vi "ArdnoFeed.vi"(0 "LINX Resource":T2={"IO"=enum."Remote", "Interface"=enum."Serial", "LINX Device Config"={"Interface"=enum."Serial", "COM Port"="COM13", "TCP Configuration"={"IP Address"="", "Port"=0}, "Device Family"=1, "Device ID"=1, "Device Name"="myRIO-1900", "TCP Ref"=refnum, "Channels"={"DI"=[0, 1, 2, 3, 4, 5, 6, 7, 8, 9, 10, 11, 12, 13, 14, 15, 16, 17, 18, 19, 20, 21, 22, 23, 24, 25, 26, 27, 28, 29, 30, 31, 32, 33, 34, 35, 36, 37, 38, 39, 40, 41, 42, 43, 44, 45, 46], "DO"=[0, 1, 2, 3, 4, 5, 6, 7, 8, 9, 10, 11, 12, 13, 14, 15, 16, 17, 18, 19, 20, 21, 22, 23, 24, 25, 26, 27, 28, 29, 30, 31, 32, 33, 34, 35, 36, 37, 38, 39, 40, 41, 42, 43, 44, 45, 46], "AI"=[0, 1, 2, 3, 4, 5, 6, 7, 8, 9, 10, 11], "AO"=[], "PWM"=[3, 5, 6, 9, 10], "QE"=[], "UART"=[0, 1], "I2C 2"=[0], "SPI"=[0], "CAN"=[], "Servo"=[], "AI Ref (V)"=0.0, "AI Resolution (Bits)"=0, "AO Ref (V)"=0.0, "AO Resolution (Bits)"=0}}}, 1 "Single / Multiring?":bool, 5 "Channel":u32, 7 "Ring":u16, 9 "Feed Cycles":i32, 11 "error in (no error)":errorcluster, 12 "All Rings":bool) -> (4 "LINX Resource out":T2, 6 "Elapsed [ms]":u32, 15 "error out":errorcluster)   [LabVIEW 2018, in "Arduino.lvlib"]
uses:
  Arduino.lvlib
  <vilib>/MakerHub/LINX/Private/Type Defs/LINX Ref.ctl
  <vilib>/MakerHub/LINX/Private/Type Defs/Platform.ctl
  <vilib>/MakerHub/LINX/Private/Type Defs/Interface.ctl
  <vilib>/MakerHub/LINX/Private/Device/Type Defs/LINX Device Config.ctl
  <vilib>/MakerHub/LINX/Private/Device/Type Defs/TCP Config.ctl
  <vilib>/MakerHub/LINX/Private/Device/Type Defs/Channels.ctl
  <vilib>/MakerHub/LINX/Public/Peripherals/Digital/Digital Write N Chans.vi
  <vilib>/MakerHub/LINX/Private/Local IO/LinxDigitalWrite.vi
  <vilib>/MakerHub/LINX/Public/Utilities/Check Channel.vi
  <vilib>/MakerHub/LINX/Private/Utilties/Generate Error.vi
  <vilib>/MakerHub/LINX/LMH-LINX.lvlib
  <vilib>/MakerHub/LINX/Private/Device/Device.lvlib
panel:
  in  "ValveManualCluster":T1
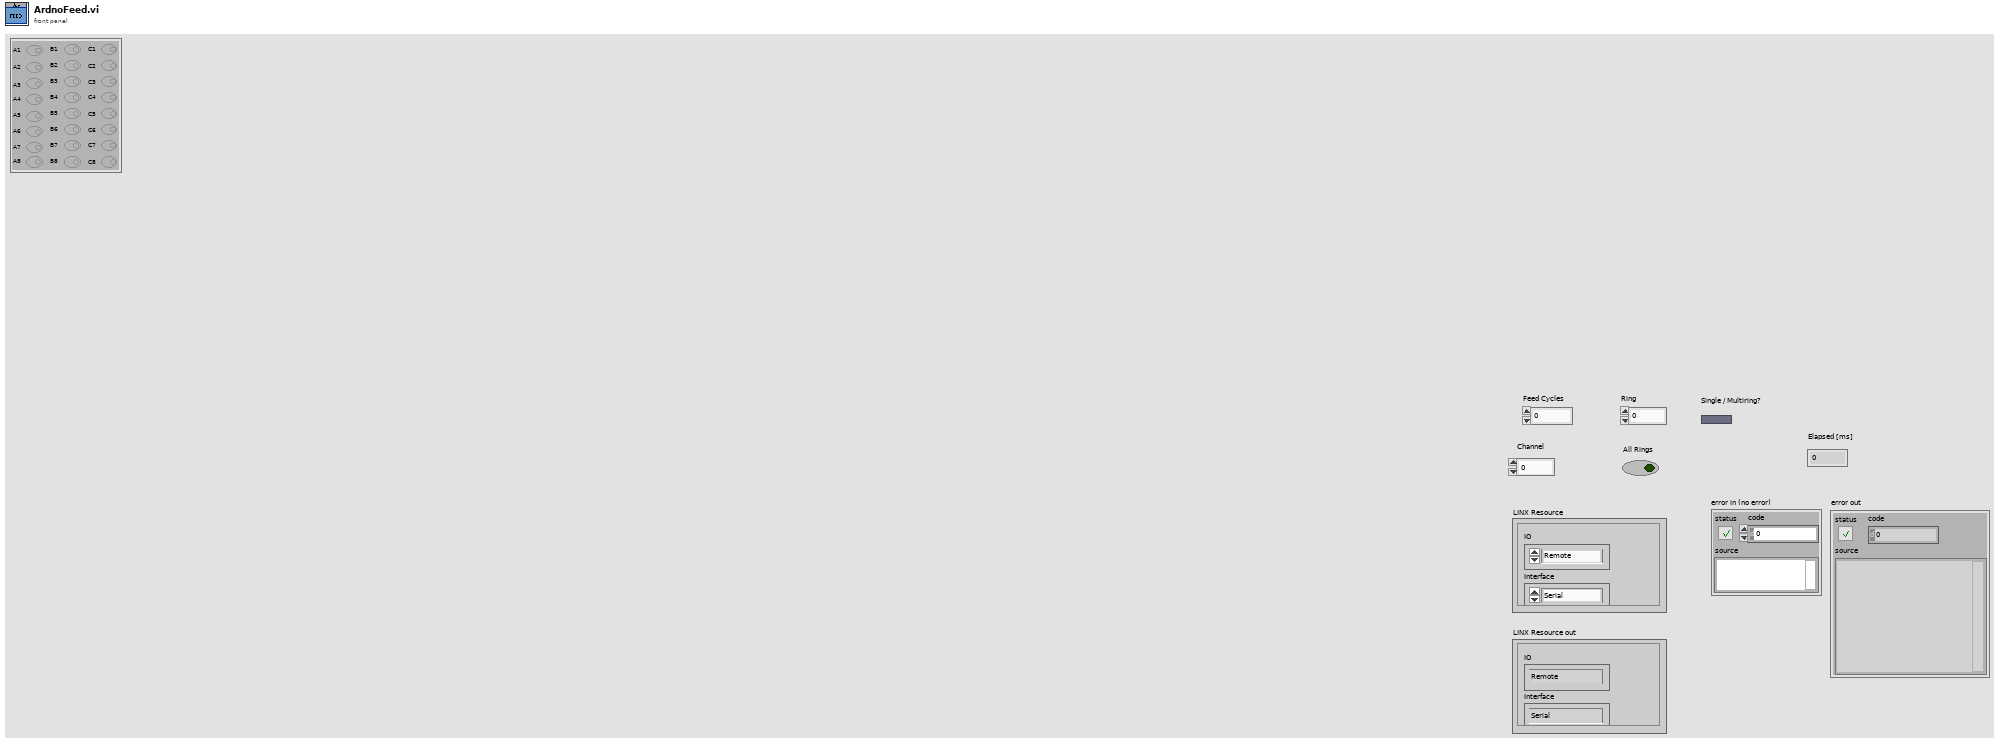
[diagram p1: front panel]
types:
  T1 = cluster{"C8":bool, "C7":bool, "C6":bool, "C5":bool, "C4":bool, "C3":bool, "C2":bool, "C1":bool, "B8":bool, "B7":bool, "B6":bool, "B5":bool, "B4":bool, "B3":bool, "B2":bool, "B1":bool, "A8":bool, "A7":bool, "A6":bool, "A5":bool, "A4":bool, "A3":bool, "A2":bool, "A1":bool}
  T2 = typedef "LMH-LINX.lvlib/LINX Ref.ctl" = cluster{"IO":T3, "Interface":T4, "LINX Device Config":T5}
  T3 = typedef "LMH-LINX.lvlib/Platform.ctl" = enum16{"Remote", "Local"}
  T4 = typedef "LMH-LINX.lvlib/Interface.ctl" = enum16{"Serial", "TCP"}
  T5 = typedef "LMH-LINX.lvlib/Device.lvlib/LINX Device Config.ctl" = cluster{"Interface":T4, "COM Port":refnum<visa-resource-name>, "TCP Configuration":T6, "Device Family":u8, "Device ID":u8, "Device Name":string, "TCP Ref":refnum<k5>, "Channels":T7}
  T6 = typedef "LMH-LINX.lvlib/Device.lvlib/TCP Config.ctl" = cluster{"IP Address":string, "Port":u16}
  T7 = typedef "LMH-LINX.lvlib/Channels.ctl" = cluster{"DI":u8[], "DO":u8[], "AI":u8[], "AO":u8[], "PWM":u8[], "QE":u8[], "UART":u8[], "I2C 2":u8[], "SPI":u8[], "CAN":u8[], "Servo":u8[], "AI Ref (V)":dbl, "AI Resolution (Bits)":u8, "AO Ref (V)":dbl, "AO Resolution (Bits)":u8}
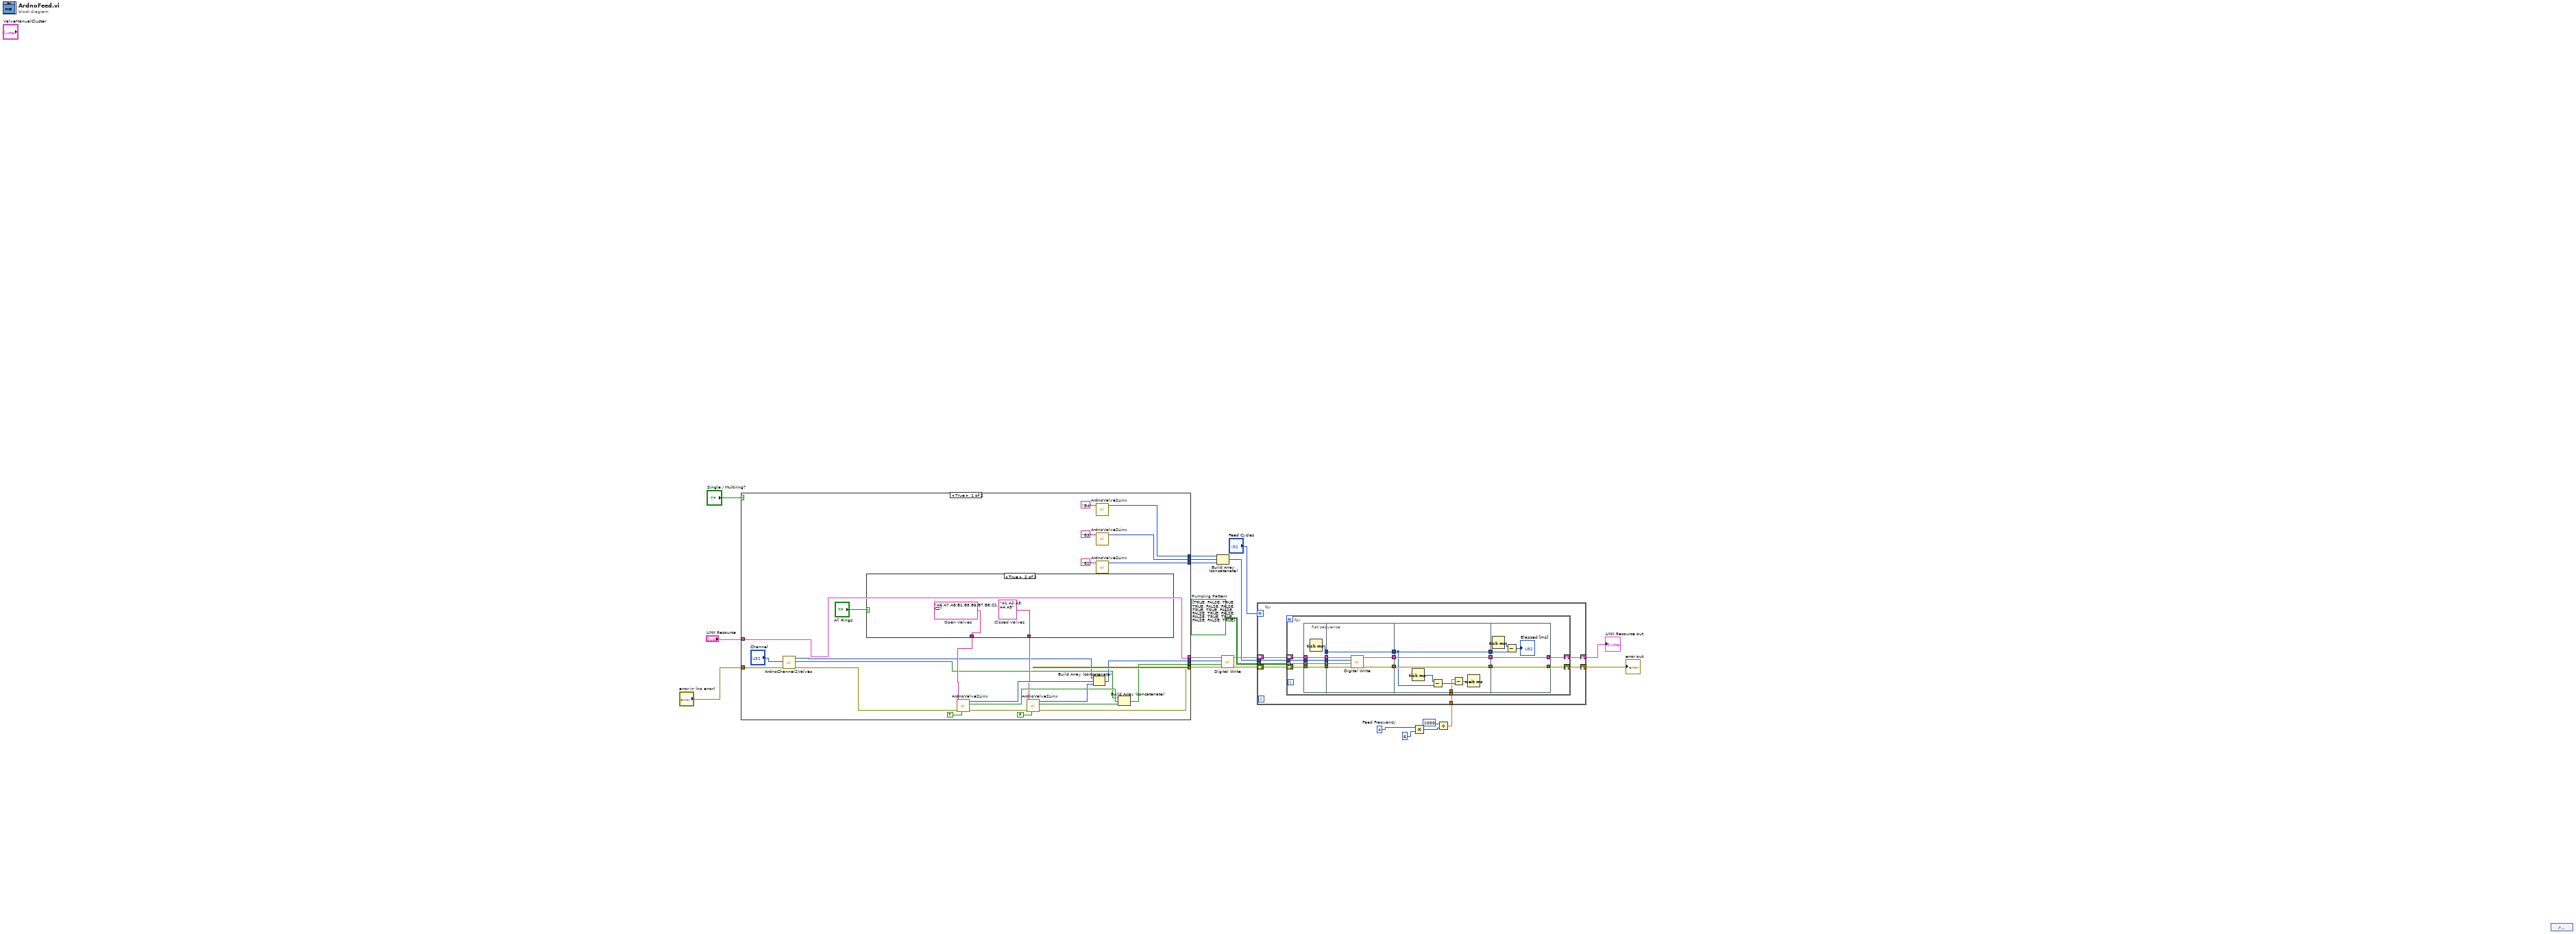
[diagram p0: block diagram]
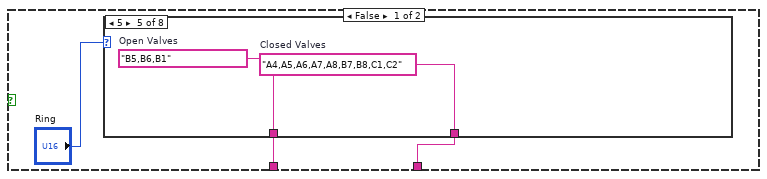
[diagram p2: hidden frame]
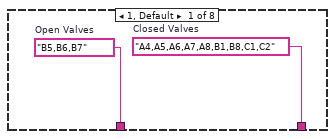
[diagram p3: hidden frame]
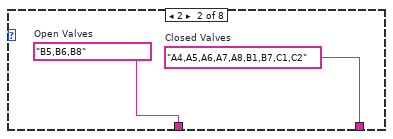
[diagram p4: hidden frame]
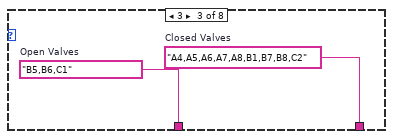
[diagram p5: hidden frame]
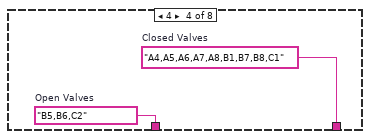
[diagram p6: hidden frame]
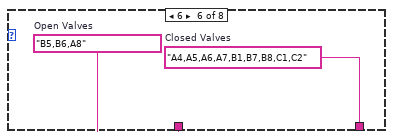
[diagram p7: hidden frame]
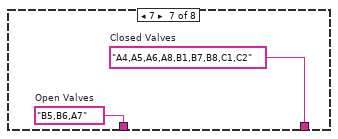
[diagram p8: hidden frame]
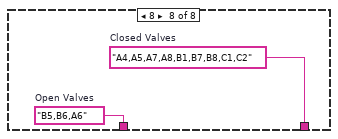
[diagram p9: hidden frame]
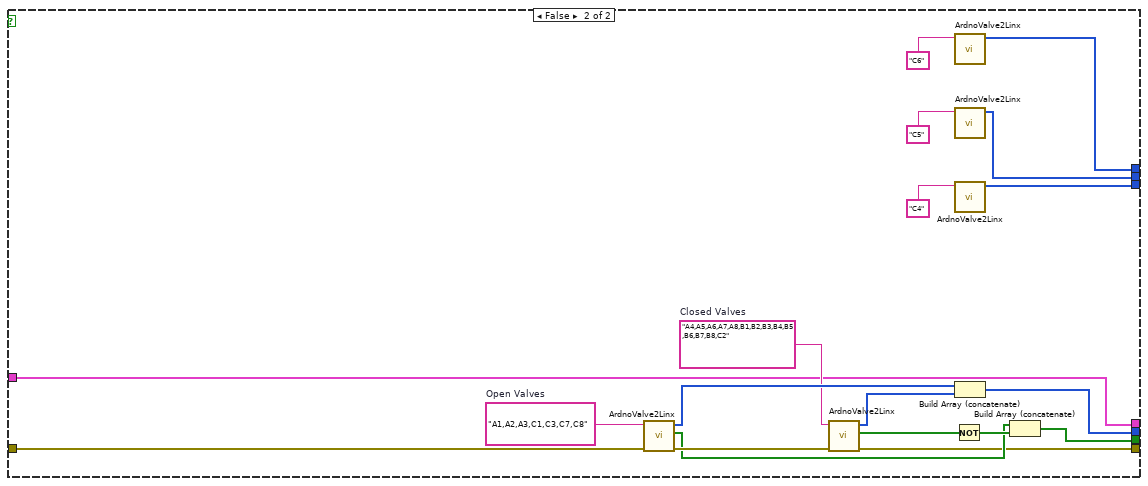
[diagram p10: hidden frame]
diagram:
  w1 = u32 4  # Feed Frequency
  w15 = bool[][] [[TRUE, FALSE, TRUE], [TRUE, FALSE, FALSE], [TRUE, TRUE, FALSE], [FALSE, TRUE, FALSE], [FALSE, TRUE, TRUE], [FALSE, FALSE, TRUE]]  # Pumping Pattern
  n1 = case shown="True" "Single / Multiring?" {
    tunnel: "error in (no error)" -> [w47 w84]
    tunnel: "LINX Resource" -> [w25 w75]
    tunnel: [w28 w74] -> w9
    tunnel: [w29 w73] -> w8
    tunnel: [w27 w72] -> w7
    tunnel: [w25 w75] -> w6
    tunnel: [w42 w71] -> w5
    tunnel: [w41 w70] -> w4
    tunnel: [w40 w69] -> w3
    frame True {
      n2 = call "ArdnoChannel2Valves.vi"("Channel"="Channel", "error in (no error)"=w47) -> ("Valve Nums"=w23:i32[], "Valve State"=w24:bool[], "error out"=w26:errorcluster)  [unwired: 6 in]
      n3 = case shown="True" "All Rings" {
        tunnel: [w49 w68] -> w31
        tunnel: [w48 w67] -> w30
        frame False {
          n4 = case shown="5" "Ring" {
            tunnel: [w52 w54 w56 w58 w60 w62 w64 w66] -> w49
            tunnel: [w51 w53 w55 w57 w59 w61 w63 w65] -> w48
            frame 1, Default {
              w51 = "A4,A5,A6,A7,A8,B1,B8,C1,C2"  # Closed Valves
              w52 = "B5,B6,B7"  # Open Valves
            }
            frame 2 {
              w53 = "A4,A5,A6,A7,A8,B1,B7,C1,C2"  # Closed Valves
              w54 = "B5,B6,B8"  # Open Valves
            }
            frame 3 {
              w55 = "A4,A5,A6,A7,A8,B1,B7,B8,C2"  # Closed Valves
              w56 = "B5,B6,C1"  # Open Valves
            }
            frame 4 {
              w57 = "A4,A5,A6,A7,A8,B1,B7,B8,C1"  # Closed Valves
              w58 = "B5,B6,C2"  # Open Valves
            }
            frame 5 {
              w59 = "A4,A5,A6,A7,A8,B7,B8,C1,C2"  # Closed Valves
              w60 = "B5,B6,B1"  # Open Valves
            }
            frame 6 {
              w61 = "A4,A5,A6,A7,B1,B7,B8,C1,C2"  # Closed Valves
              w62 = "B5,B6,A8"  # Open Valves
            }
            frame 7 {
              w63 = "A4,A5,A6,A8,B1,B7,B8,C1,C2"  # Closed Valves
              w64 = "B5,B6,A7"  # Open Valves
            }
            frame 8 {
              w65 = "A4,A5,A7,A8,B1,B7,B8,C1,C2"  # Closed Valves
              w66 = "B5,B6,A6"  # Open Valves
            }
          }
        }
        frame True {
          w67 = "A1,A2,A3,A4,A5"  # Closed Valves
          w68 = "A6,A7,A8,B1,B5,B6,B7,B8,C1,C2"  # Open Valves
        }
      }
      n5 = call "ArdnoValve2Linx.vi"("Open?"=TRUE, "error in (no error)"=w26, "Valve (A1-C8),\n comma separated"=w31) -> ("error out"=w32:errorcluster, "Closed State"=w33:bool[], "Linx Port"=w34:i32[])  [unwired: 6 in]
      n6 = call "ArdnoValve2Linx.vi"("Open?"=FALSE, "error in (no error)"=w32, "Valve (A1-C8),\n comma separated"=w30) -> ("error out"=w27:errorcluster, "Closed State"=w36:bool[], "Linx Port"=w35:i32[])  [unwired: 6 in]
      n7 = Build Array (concatenate)(w23, w34, w35) -> (w28:i32[])
      n8 = call "ArdnoValve2Linx.vi"("Valve (A1-C8),\n comma separated"="B4") -> ("Linx Port"=w42:i32[])  [unwired: 8 in, 2 out]
      n9 = call "ArdnoValve2Linx.vi"("Valve (A1-C8),\n comma separated"="B3") -> ("Linx Port"=w41:i32[])  [unwired: 8 in, 2 out]
      n10 = call "ArdnoValve2Linx.vi"("Valve (A1-C8),\n comma separated"="B2") -> ("Linx Port"=w40:i32[])  [unwired: 8 in, 2 out]
      n11 = Build Array (concatenate)(w24, w33, w36) -> (w29:bool[])
    }
    frame False {
      w77 = "A4,A5,A6,A7,A8,B1,B2,B3,B4,B5,B6,B7,B8,C2"  # Closed Valves
      w76 = "A1,A2,A3,C1,C3,C7,C8"  # Open Valves
      n12 = call "ArdnoValve2Linx.vi"("error in (no error)"=w84, "Valve (A1-C8),\n comma separated"=w76) -> ("error out"=w83:errorcluster, "Closed State"=w81:bool[], "Linx Port"=w80:i32[])  [unwired: 7 in]
      n13 = call "ArdnoValve2Linx.vi"("error in (no error)"=w83, "Valve (A1-C8),\n comma separated"=w77) -> ("error out"=w72:errorcluster, "Closed State"=w78:bool[], "Linx Port"=w79:i32[])  [unwired: 7 in]
      n14 = Not(x=w78) -> (.not. x?=w82:bool[])
      n15 = call "ArdnoValve2Linx.vi"("Valve (A1-C8),\n comma separated"="C6") -> ("Linx Port"=w71:i32[])  [unwired: 8 in, 2 out]
      n16 = call "ArdnoValve2Linx.vi"("Valve (A1-C8),\n comma separated"="C5") -> ("Linx Port"=w70:i32[])  [unwired: 8 in, 2 out]
      n17 = call "ArdnoValve2Linx.vi"("Valve (A1-C8),\n comma separated"="C4") -> ("Linx Port"=w69:i32[])  [unwired: 8 in, 2 out]
      n18 = Build Array (concatenate)(w80, w79) -> (w74:i32[])
      n19 = Build Array (concatenate)(w81, w82) -> (w73:bool[])
    }
  }
  n20 = Build Array (concatenate)(w5, w4, w3) -> (w14:i32[])
  n21 = call-poly <vilib>:"Digital Write.vi"("Error In"=w7, "Values"=w8, "DO Channels"=w9, "LINX Resource"=w6) -> ("Error Out"=w13:errorcluster, "LINX Resource"=w12:T2)  [unwired: 6 in]
  n22 = Multiply(x=w1, y=u32 6) -> (x*y=w16:u32)
  n23 = Divide(x=u32 1000, y=w16) -> (x/y=w17:dbl)
  n24 = for {
    N: "Feed Cycles" -> [_]
    tunnel: w14 -> [w92]
    tunnel: w15 -> [w91]
    shift-right: [w90] -> w11
    shift-left: w12 -> [w94]
    shift-right: [w89] -> w10
    shift-left: w13 -> [w93]
    tunnel: w17 -> [w88]
    n25 = for {
      tunnel: w91 -> [w107] mode=indexing
      tunnel: w92 -> [w110]
      shift-right: [w109] -> w90
      shift-left: w94 -> [w112]
      shift-right: [w108] -> w89
      shift-left: w93 -> [w111]
      tunnel: w88 -> [w98]
      n26 = flat-sequence {
        tunnel: w107 -> [w114]
        tunnel: w110 -> [w115]
        tunnel: w111 -> [w116]
        tunnel: w112 -> [w117]
        tunnel: [w117] -> w106
        tunnel: [w116] -> w105
        tunnel: [w115] -> w104
        tunnel: [w114] -> w103
        tunnel: [w113] -> w102
        tunnel: [w121] -> w97
        tunnel: [w120] -> w96
        tunnel: w106 -> [w124]
        tunnel: w105 -> [w123]
        tunnel: w104 -> [w122]
        tunnel: w103 -> [w119]
        tunnel: w102 -> [w118]
        tunnel: [w118] -> w95
        tunnel: w97 -> [w131]
        tunnel: w96 -> [w130]
        tunnel: w95 -> [w128]
        tunnel: [w131] -> w101
        tunnel: [w130] -> w100
        tunnel: [w128] -> w99
        tunnel: w98 -> [w125]
        tunnel: [w135] -> w108
        tunnel: [w136] -> w109
        tunnel: w101 -> [w136]
        tunnel: w100 -> [w135]
        tunnel: w99 -> [w132]
        frame #0 {
          n27 = Tick Count (ms)() -> (millisecond timer value=w113:u32)
        }
        frame #1 {
          n28 = call-poly <vilib>:"Digital Write.vi"("Error In"=w123, "Values"=w119, "DO Channels"=w122, "LINX Resource"=w124) -> ("Error Out"=w120:errorcluster, "LINX Resource"=w121:T2)  [unwired: 6 in]
        }
        frame #2 {
          n29 = Tick Count (ms)() -> (millisecond timer value=w129:u32)
          n30 = Subtract(x=w129, y=w128) -> (x-y=w127:u32)
          n31 = Subtract(x=w125, y=w127) -> (x-y=w126:dbl)
          n32 = Wait (ms)(milliseconds to wait=w126) -> ()  [unwired: 1 out]
        }
        frame #3 {
          n33 = Tick Count (ms)() -> (millisecond timer value=w133:u32)
          n34 = Subtract(x=w133, y=w132) -> (x-y=→"Elapsed [ms]":u32)
        }
      }
    }
  }
  "error out" <- w10
  "LINX Resource out" <- w11
  n35 = control-ref of="ValveManualCluster"() -> ()  [unwired: 1 out]
